vi "subvi.vi"() -> ()   [LabVIEW 2020]
uses:
  <vilib>/ErrorRing/Error Ring.xnode
panel:
  in  "Formato":string(combo)
  in  "Nombre":string
  in  "Direccion":path
  out "Array":dbl[](array[slide]) scale=0.0..100.0
  in  "N":i32
  in  "Lmin":dbl
  in  "Lmax":dbl
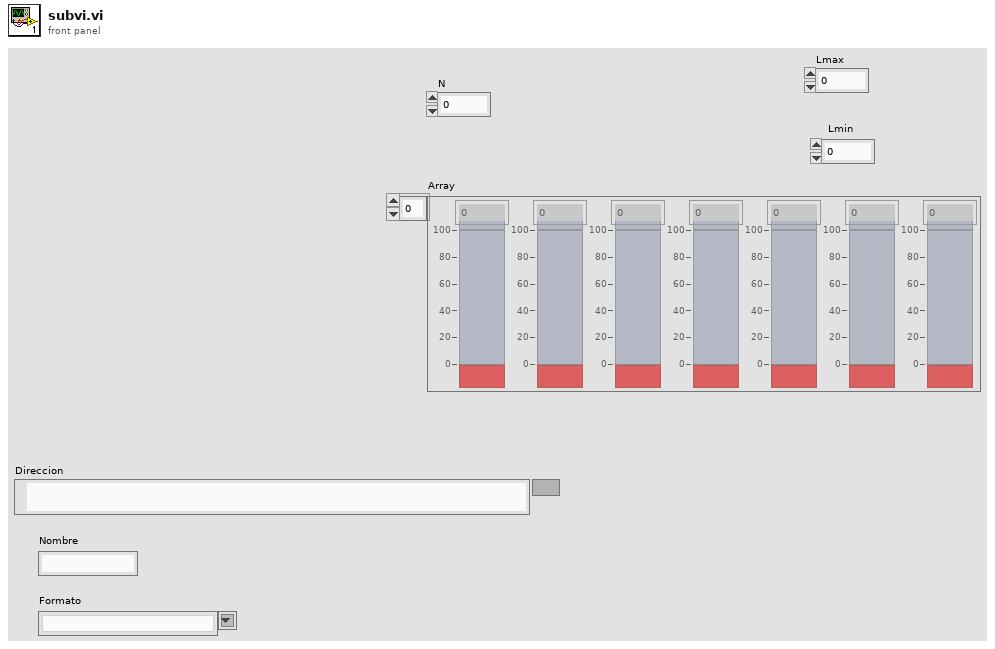
[diagram p1: front panel]
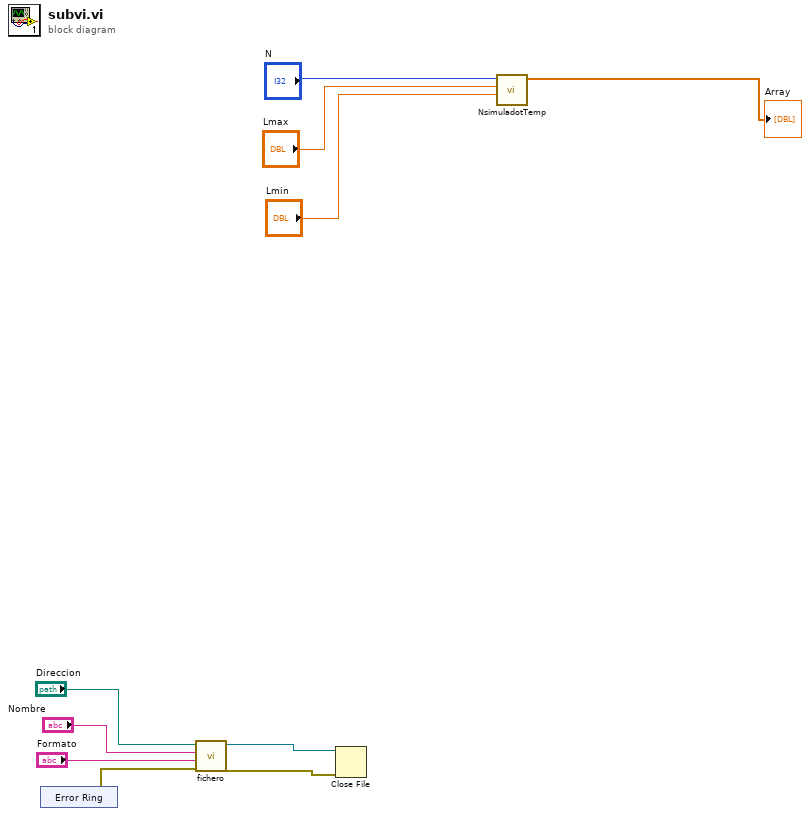
[diagram p0: block diagram]
diagram:
  n1 = xnode "Error Ring"() -> ("error out"=w3:errorcluster)
  n2 = call "fichero.vi"("error in (no error)"=w3, "Formato"="Formato", "Nombre"="Nombre", "Direccion"="Direccion") -> ("error out"=w1:errorcluster, "Byte Stream File out"=w2:refnum<file>)  [unwired: 6 in]
  n3 = Close File(refnum=w2, error in=w1) -> ()  [unwired: 2 out]
  n4 = call "NsimuladotTemp.vi"("Lmin"="Lmin", "Lmax"="Lmax", "N"="N") -> ("Array"=→"Array":dbl[])  [unwired: 8 in]
